vi "TransferData Example.vi"() -> ()   [LabVIEW 2015]
uses:
  Engine/SubVIs/GMLAN/_SubVIs/SecurityAccess_requestSeed_SubFunctions.ctl
  Engine/SubVIs/GMLAN/_SubVIs/TransferData_SubFunction.ctl
  <vilib>/Automotive Diagnostic Command Set/Diagnostic Transport.llb/Property ID.ctl
  Engine/SubVIs/GMLAN/_SubVIs/DisableNormalCommunication_Parameter.ctl
  Engine/SubVIs/GMLAN/_SubVIs/ProgrammingMode_SubFunction.ctl
  <vilib>/Automotive Diagnostic Command Set/Diagnostic Transport.llb/Transport Protocol Selector.ctl
  Engine/SubVIs/GMLAN/_SubVIs/TesterPresent_Parameter.ctl
  Engine/SubVIs/GMLAN/_SubVIs/SecurityAccess_requestSeed.vi
  Engine/SubVIs/GMLAN/_SubVIs/SecurityAccess_sendKey.vi
  Engine/SubVIs/GMLAN/Utilities/GMLAN Service Broadcast.vi
  <vilib>/Automotive Diagnostic Command Set/Diagnostic Transport.llb/Diag Globals.vi
  <vilib>/Automotive Diagnostic Command Set/Diagnostic Transport.llb/Diagnostic Service Send.vi
  <vilib>/Automotive Diagnostic Command Set/Diagnostic Transport.llb/Diagnostic Response Recv.vi
  <vilib>/Automotive Diagnostic Command Set/Diagnostic Transport.llb/Apply Diagnostic Error.vi
  <vilib>/Automotive Diagnostic Command Set/Diagnostic Transport.llb/Diagnostic Service.vi
  <vilib>/Automotive Diagnostic Command Set/Diagnostic Transport.llb/Apply Success Failure Error.vi
  <vilib>/addons/Automotive Diagnostic Command Set/NI_Automotive Diagnostic Command Set.lvlib
  Engine/SubVIs/GMLAN/GMLAN.lvlib
panel:
  in  "startingAddress Length":enum8{"Two", "Three", "Four"}(ring)
  in  "startingAddress":u32
  in  "subFuntion":T1 items=["download"=0, "downloadAndExecuteOrExecute"=128]
  in  "dataRecord":u8[](array[numeric]) format="%.0x"
  in  "dataFormatIdentifier":u8 format="%.0b"
  in  "unCompressedMemorySize":u32
  in  "unCompressedMemorySize Length":enum8{"Two", "Three", "Four"}(ring)
  out "stopped?":bool=TRUE
  out "error IO":errorcluster
  in  "subFunction":T2=1 items=["SPSrequestSeed"=1, "DevCtrlrequestSeed"=3]
  in  "Transmit ID":u32=2016 format="%.0x"
  in  "Receive ID":u32=2024 format="%.0x"
  in  "Baudrate":u32=500000
  in  "CAN Interface":string(combo)="CAN1"
  in  "HW select":u16(ring) items=["NI-XNET", "NI-CAN"]
  in  "UUDT Receive ID":u32=1512 format="%.0x"
  # "Initial Parameters"
  # "Service x27"
  # "Service x34"
  # "Service x34"
  # "Status"
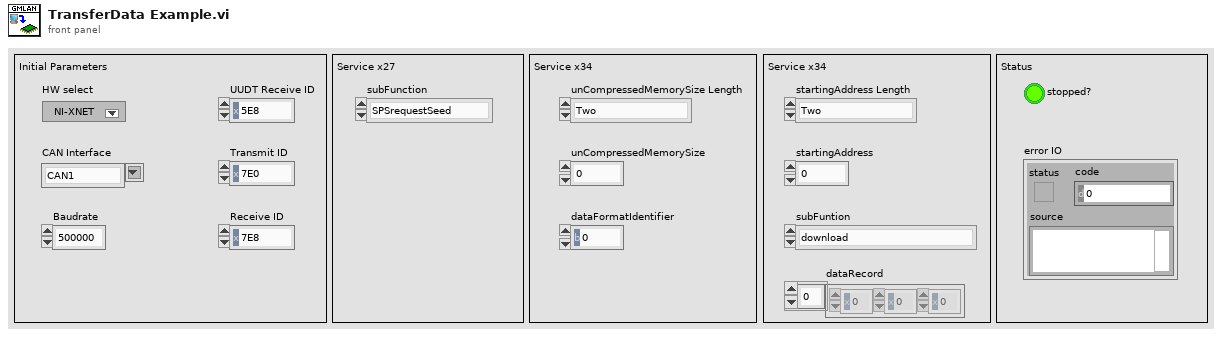
[diagram p1: front panel]
types:
  T1 = typedef "GMLAN.lvlib/TransferData_SubFunction.ctl" = u8
  T2 = typedef "GMLAN.lvlib/SecurityAccess_requestSeed_SubFunctions.ctl" = u8
  T3 = typedef "GMLAN.lvlib/ProgrammingMode_SubFunction.ctl" = u8
  T4 = typedef "GMLAN.lvlib/DisableNormalCommunication_Parameter.ctl" = enum8{"SpecificECU", "EntireNetwork"}
  T5 = typedef "NI_Automotive Diagnostic Command Set.lvlib/Property ID.ctl" = enum16{"Timeout Diag Command", "Timeout FC (Bs)", "Timeout CF (Cr)", "Receive Block Size (BS)", "Wait Time CF (STmin)", "Max Wait Frames (N_WFTmax)", "Wait Frames to Send (N_WAIT)", "Time between Waits (T_W)", "Fill CAN Frames", "Fill Byte", "Invalid Response as Error", "Max RspPending Count", "VWTP Command Timeout", "STmin", "P2min", "Termination"}
  T6 = typedef "NI_Automotive Diagnostic Command Set.lvlib/Transport Protocol Selector.ctl" = enum16{"ISO TP - Normal Mode", "ISO TP - Mixed Mode", "VW TP 2.0", "Diagnostics on IP", "ISO TP LIN"}
  T7 = typedef "NI_Automotive Diagnostic Command Set.lvlib/Diag Reference.ctl" = cluster{"Diag CAN Handle":u32, "Transport Protocol":T6, "Receive Address Extension":u8, "Transmit Address Extension":u8, "Receive CAN Id":u32, "Transmit CAN Id":u32, "Diag CAN Queue":refnum<queue>, "Log Frames ?":bool, "My TP Address":u8, "Other TP Address":u8, "T1":u16, "T2":u16, "T3":u16, "T4":u16, "Tx SN":u8, "Block Size":u8, "Rx SN":u8, "VW TP Initialized?":bool, "Tx block no":u8, "baud rate":u32, "Interface":string, "Channel Diag CAN Handle":u32, "UDP Connection ID":refnum<k16>, "TCP Connection ID":refnum<k5>, "Target IP Addr":u32, "Source Address":u16, "Target Address":u16, "Send Header NACK?":bool, "DLL Handle":u32, "NAD":u8, "Time Stamp read first":dbl, "Time Stamp read last":dbl, "Time Stamp write first":dbl, "Time Stamp write last":dbl, "Time Stamp write":dbl, "Time Stamp read":dbl}
  T8 = typedef "GMLAN.lvlib/TesterPresent_Parameter.ctl" = enum8{"SpecificECU", "EntireNetwork"}
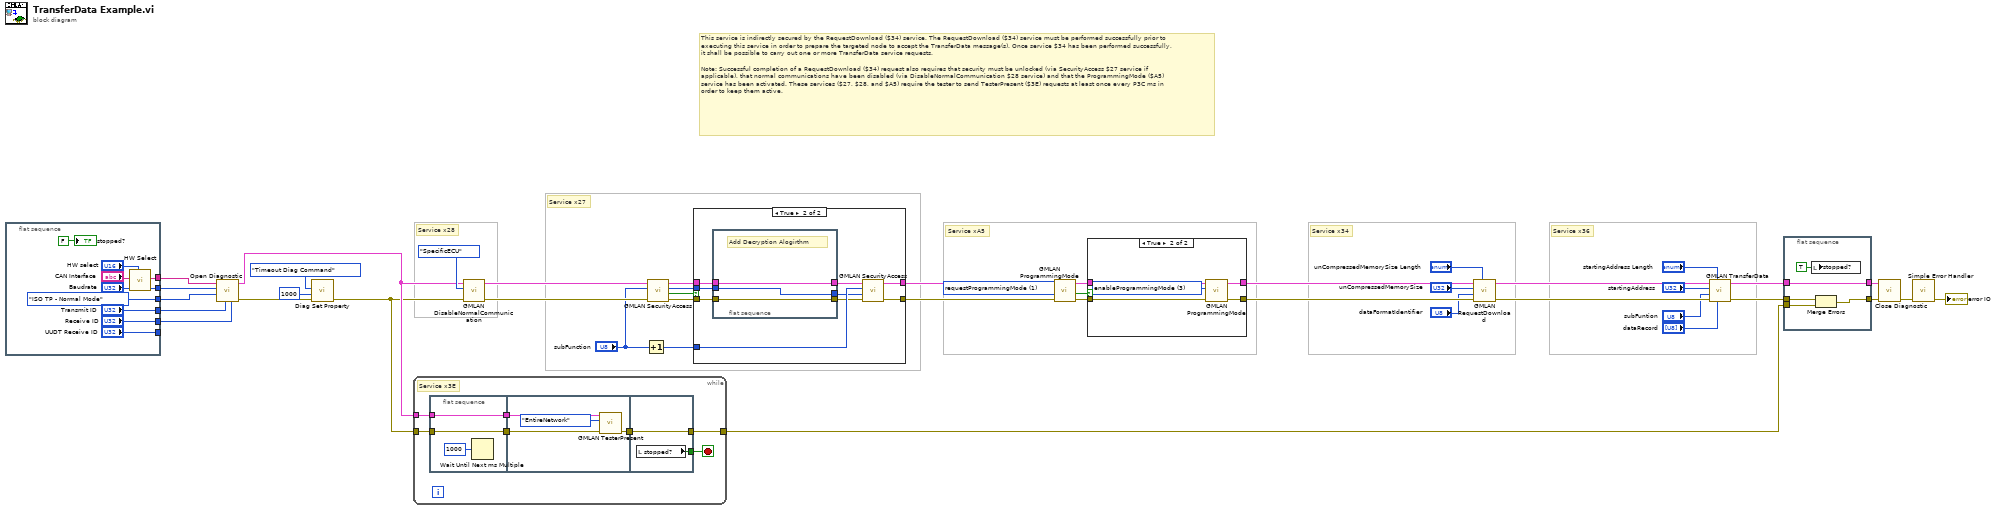
[diagram p0: block diagram]
diagram:
  w21 = T3 1 items=["requestProgrammingMode"=1, "requestProgrammingMode_HighSpeed"=2, "enableProgrammingMode"=3] ("subFunction")
  # "This service is indirectly secured by the RequestDownload ($34) service. The RequestDownload ($34) service must be performed successfully prior to executing this service in order to prepare the targeted node to accept the TransferData message(s). Once service $34 has been performed successfully, it shall be possible to carry out one or more TransferData service requests.\n\nNote: Successful completion of a RequestDownload ($34) request also requires that security must be unlocked (via SecurityAccess $27 service if applicable), that normal communications have been disabled (via DisableNormalCommunication $28 service) and that the ProgrammingMode ($A5) service has been activated. These services ($27, $28, and $A5) require the tester to send TesterPresent ($3E) requests at least once every P3C ms in order to keep them active."
  # "Service x36"
  # "Service x34"
  # "Service x28"
  # "Service x27"
  # "Service xA5"
  n1 = flat-sequence {
    tunnel: [w52] -> w43
    tunnel: ["Baudrate"] -> w36
    tunnel: [Transport_Protocol_Selector."ISO TP - Normal Mode" ("Transport Protocol")] -> w42
    tunnel: ["Transmit ID"] -> w41
    tunnel: ["Receive ID"] -> w40
    tunnel: ["UUDT Receive ID"] -> _
    frame #0 {
      n2 = call "HW Select.vi"("HW select"="HW select", "CAN port"="CAN Interface") -> ("CAN port out"=w52:string)  [unwired: 9 in]
      "stopped?" <- FALSE ("stopped?")
    }
  }
  n3 = call <vilib>:"Open Diagnostic.vi"("Receive ID"=w40, "Transmit ID"=w41, "Transport Protocol"=w42, "Baud Rate"=w36, "CAN Interface"=w43) -> ("error out"=w39:errorcluster, "diag ref out"=w25:T7)  [unwired: 1 in, 4 out]
  n4 = call <vilib>:"Diag Set Property.vi"("error in (no error)"=w39, "property value"=u32 1000, "property ID"=Property_ID."Timeout Diag Command") -> ("error out"=w24:errorcluster)  [unwired: 7 in, 1 out]
  n5 = while {
    tunnel: w25 -> [w59]
    tunnel: w24 -> [w57]
    tunnel: [w54] -> w4
    stop <- w55 stop-if-true
    # "Service x3E"
    n6 = flat-sequence {
      tunnel: w59 -> [w61]
      tunnel: [w61] -> w58
      tunnel: w57 -> [w60]
      tunnel: [w60] -> w56
      tunnel: w58 -> [w66]
      tunnel: w56 -> [w65]
      tunnel: [w63] -> w53
      tunnel: [w68] -> w55
      tunnel: [w67] -> w54
      tunnel: w53 -> [w67]
      frame #0 {
        n7 = Wait Until Next ms Multiple(millisecond multiple=u32 1000) -> ()  [unwired: 1 out]
      }
      frame #1 {
        n8 = call "GMLAN TesterPresent.vi"("error in (no error)"=w65, "Parameter"=TesterPresent_Parameter."EntireNetwork", "diag ref in"=w66) -> ("error out"=w63:errorcluster)  [unwired: 6 in, 2 out]
      }
      frame #2 {
        n9 = local read "stopped?"() -> (w68:bool)
      }
    }
  }
  n10 = call "GMLAN DisableNormalCommunication.vi"("error in (no error)"=w24, "Parameter"=DisableNormalCommunication_Parameter."SpecificECU", "diag ref in"=w25) -> ("error out"=w28:errorcluster, "diag ref out"=w27:T7)  [unwired: 6 in, 1 out]
  n11 = Increment(x="subFunction") -> (x+1=w35:T2)
  n12 = call-poly "GMLAN SecurityAccess.vi"("error in (no error)"=w28, "subFunction"="subFunction", "diag ref in"=w27) -> ("error out"=w34:errorcluster, "success?"=w31:bool, "SecuritySeed"=w32:u16, "diag ref out"=w33:T7)  [unwired: 5 in]
  n13 = case shown="True" w31 {
    tunnel: w35 -> [_ w79]
    tunnel: w34 -> [w70 w77]
    tunnel: w33 -> [w69 w75]
    tunnel: w32 -> [_ w74]
    tunnel: [w70 w73] -> w23
    tunnel: [w69 w72] -> w22
    frame False {
    }
    frame True {
      n14 = flat-sequence {
        tunnel: [w82] -> w78
        tunnel: w77 -> [w82]
        tunnel: [w81] -> w76
        tunnel: w75 -> [w81]
        tunnel: [w80] -> w71
        tunnel: w74 -> [w80]
        frame #0 {
          # "Add Decryption Alogirthm"
        }
      }
      n15 = call-poly "GMLAN SecurityAccess.vi"("error in (no error)"=w78, "SecuritySeed"=w71, "subFunction"=w79, "diag ref in"=w76) -> ("error out"=w73:errorcluster, "diag ref out"=w72:T7)  [unwired: 5 in, 1 out]
    }
  }
  n16 = call "GMLAN ProgrammingMode.vi"("error in (no error)"=w23, "subFunction"=w21, "diag ref in"=w22) -> ("error out"=w19:errorcluster, "success?"=w20:bool, "diag ref out"=w18:T7)  [unwired: 6 in]
  n17 = case shown="True" w20 {
    tunnel: w19 -> [w83 w89]
    tunnel: w18 -> [w84 w88]
    tunnel: [w83 w86] -> w17
    tunnel: [w84 w85] -> w16
    frame False {
    }
    frame True {
      w87 = T3 3 items=["requestProgrammingMode"=1, "requestProgrammingMode_HighSpeed"=2, "enableProgrammingMode"=3] ("subFunction")
      n18 = call "GMLAN ProgrammingMode.vi"("error in (no error)"=w89, "subFunction"=w87, "diag ref in"=w88) -> ("error out"=w86:errorcluster, "diag ref out"=w85:T7)  [unwired: 6 in, 1 out]
    }
  }
  n19 = call "GMLAN RequestDownload.vi"("unCompressedMemorySize Length"="unCompressedMemorySize Length", "error in (no error)"=w17, "dataFormatIdentifier"="dataFormatIdentifier", "unCompressedMemorySize"="unCompressedMemorySize", "diag ref in"=w16) -> ("error out"=w12:errorcluster, "diag ref out"=w11:T7)  [unwired: 4 in, 1 out]
  n20 = call "GMLAN TransferData.vi"("dataRecord"="dataRecord", "startingAddress Length"="startingAddress Length", "error in (no error)"=w12, "subFuntion"="subFuntion", "startingAddress"="startingAddress", "diag ref in"=w11) -> ("error out"=w5:errorcluster, "diag ref out"=w6:T7)  [unwired: 3 in, 1 out]
  n21 = flat-sequence {
    tunnel: w6 -> [w90]
    tunnel: w5 -> [w93]
    tunnel: w4 -> [w92]
    tunnel: [w91] -> w3
    tunnel: [w90] -> w2
    frame #0 {
      n22 = local write "stopped?"(TRUE ("stopped?")) -> ()
      n23 = Merge Errors(w93, w92) -> (w91:errorcluster)
    }
  }
  n24 = call <vilib>:"Close Diagnostic.vi"("error in (no error)"=w3, "diag ref in"=w2) -> ("error out"=w29:errorcluster)  [unwired: 9 out]
  n25 = call <vilib>:"Simple Error Handler.vi"("error in (no error)"=w29) -> ("error out"=→"error IO":errorcluster)  [unwired: 1 in, 7 out]
